vi "List.Fields.All.vi"(3 "Enum":i32) -> (1 "String":string)   [LabVIEW 2013]
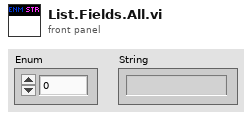
[diagram p1: front panel]
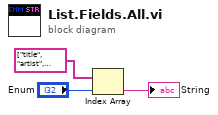
[diagram p0: block diagram]
diagram:
  n1 = Index Array(array=string[] ["title", "artist", "albumartist", "genre", "year", "rating", "album", "track", "duration", "comment", "lyrics", "musicbrainztrackid", "musicbrainzartistid", "musicbrainzalbumid", "musicbrainzalbumartistid", "playcount", "fanart", "director", "trailer", "tagline", "plot", "plotoutline", "originaltitle", "lastplayed", "writer", "studio", "mpaa", "cast", "country", "imdbnumber", "premiered", "productioncode", "runtime", "set", "showlink", "streamdetails", "top250", "votes", "firstaired", "season", "episode", "showtitle", "thumbnail", "file", "resume", "artistid", "albumid", "tvshowid", "setid", "watchedepisodes", "disc", "tag", "art", "genreid", "displayartist", "albumartistid", "description", "theme", "mood", "style", "albumlabel", "sorttitle", "episodeguide", "uniqueid", "dateadded", "channel", "channeltype", "hidden", "locked", "channelnumber", "starttime", "endtime"], index="Enum") -> (element=→"String":string)
